vi "DI sensor handling full_ext.vi"(0 "DI":bool, 1 "SOURCE":u32=1 max=2 step=1, 2 "SOURCE_ALLOW":bool, 3 "DI2":bool, 4 "control":cluster{"invert":dbl, "time_const":dbl}={"invert"=1.0, "time_const"=100.0} {"time_const" min=1.0 max=100000.0 step=1.0}, 6 "initialise":bool, 7 "DI sensor handling full reg old":T2 {"RS32 Q" format="%x"}, 8 "connect":bool) -> (13 "DI sensor handling full reg":T1 {"RS32 Q" format="%x"}, 14 "DIOUT":bool caption="PVOUT", 15 "SOURCEOUT":u32=1 max=2 step=1, 16 "STATE":T3, 17 "block":u32 format="%09b", 19 "ALRSTATE":errorcluster)   [LabVIEW 2019, in "Inputs.lvlib"]
uses:
  Inputs.lvlib
  Ctl/Parameter State.ctl
  Ctl/Sensor alarm.ctl
  Ctl/Sensor state.ctl
  Trigers/RS_ext.vi
  Logik/Logik.lvlib
  Trigers/Triggers.lvlib
  Timer Delay/Timers.lvlib
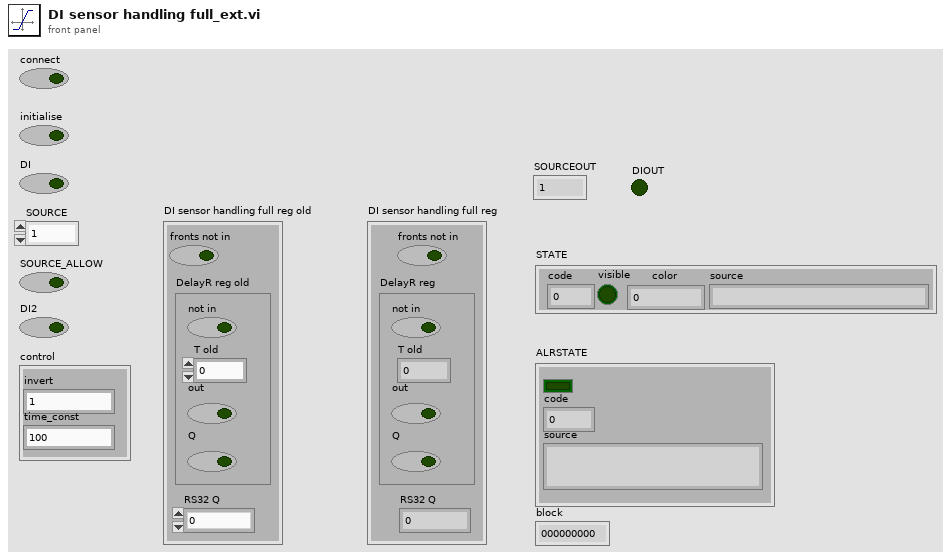
[diagram p1: front panel]
types:
  T1 = cluster{"fronts not in":bool, "DelayR reg":cluster{"not in":bool, "T old":u32, "out":bool, "Q":bool}, "RS32 Q":u32}
  T2 = cluster{"fronts not in":bool, "DelayR reg old":cluster{"not in":bool, "T old":u32, "out":bool, "Q":bool}, "RS32 Q":u32}
  T3 = typedef "Inputs.lvlib/Parameter State.ctl" = cluster{"code":i32, "visible":bool, "color":u32, "source":string}
  T4 = typedef "Inputs.lvlib/Sensor alarm.ctl" = cluster{"source":string, "color":u32, "visible":bool}[]
  T5 = typedef "Inputs.lvlib/Sensor state.ctl" = cluster{"source":string, "color":u32, "visible":bool}[]
  T6 = cluster{"not in":bool, "T old":u32, "out":bool, "Q":bool}
  T7 = cluster{"source":string, "color":u32, "visible":bool}
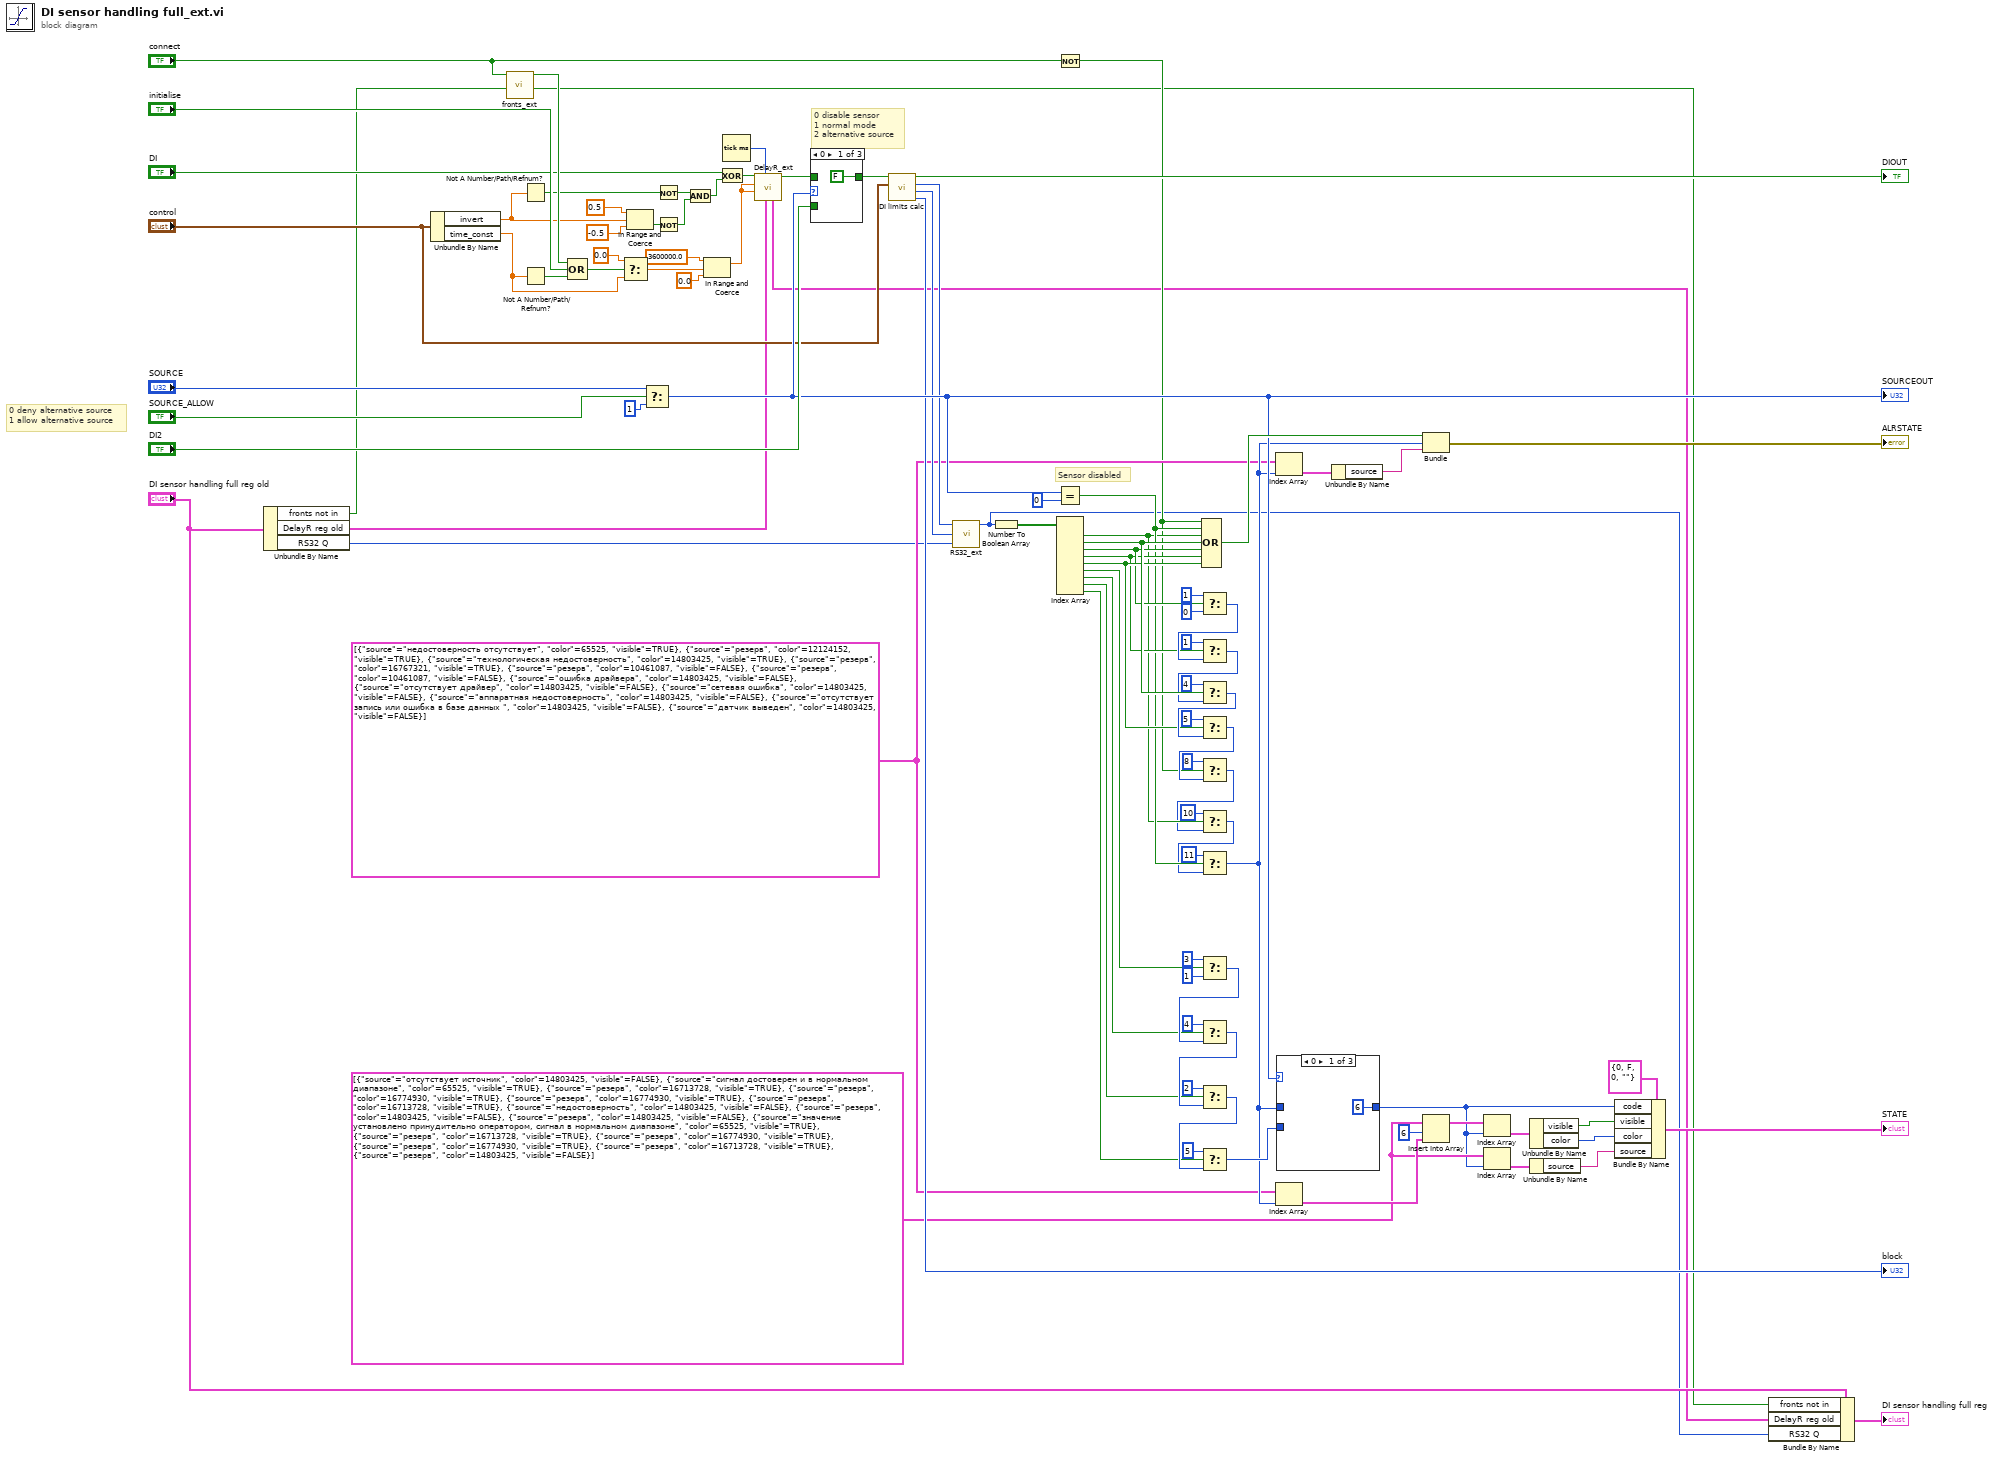
[diagram p0: block diagram]
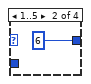
[diagram p5: hidden frame]
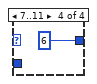
[diagram p7: hidden frame]
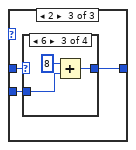
[diagram p8: hidden frame]
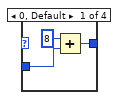
[diagram p9: hidden frame]
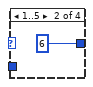
[diagram p10: hidden frame]
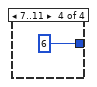
[diagram p11: hidden frame]
diagram:
  w39 = T4 [{"source"="недостоверность отсутствует", "color"=65525, "visible"=TRUE}, {"source"="резерв", "color"=12124152, "visible"=TRUE}, {"source"="технологическая недостоверность", "color"=14803425, "visible"=TRUE}, {"source"="резерв", "color"=16767321, "visible"=TRUE}, {"source"="резерв", "color"=10461087, "visible"=FALSE}, {"source"="резерв", "color"=10461087, "visible"=FALSE}, {"source"="ошибка драйвера", "color"=14803425, "visible"=FALSE}, {"source"="отсутствует драйвер", "color"=14803425, "visible"=FALSE}, {"source"="сетевая ошибка", "color"=14803425, "visible"=FALSE}, {"source"="аппаратная недостоверность", "color"=14803425, "visible"=FALSE}, {"source"="отсутствует запись или ошибка в базе данных ", "color"=14803425, "visible"=FALSE}, {"source"="датчик выведен", "color"=14803425, "visible"=FALSE}]
  w47 = T5 [{"source"="отсутствует источник", "color"=14803425, "visible"=FALSE}, {"source"="сигнал достоверен и в нормальном диапазоне", "color"=65525, "visible"=TRUE}, {"source"="резерв", "color"=16713728, "visible"=TRUE}, {"source"="резерв", "color"=16774930, "visible"=TRUE}, {"source"="резерв", "color"=16774930, "visible"=TRUE}, {"source"="резерв", "color"=16713728, "visible"=TRUE}, {"source"="недостоверность", "color"=14803425, "visible"=FALSE}, {"source"="резерв", "color"=14803425, "visible"=FALSE}, {"source"="резерв", "color"=14803425, "visible"=FALSE}, {"source"="значение установлено принудительно оператором, сигнал в нормальном диапазоне", "color"=65525, "visible"=TRUE}, {"source"="резерв", "color"=16713728, "visible"=TRUE}, {"source"="резерв", "color"=16774930, "visible"=TRUE}, {"source"="резерв", "color"=16774930, "visible"=TRUE}, {"source"="резерв", "color"=16713728, "visible"=TRUE}, {"source"="резерв", "color"=14803425, "visible"=FALSE}]
  # "Sensor disabled"
  # "0 disable sensor\n1 normal mode\n2 alternative source"
  # "0 deny alternative source\n1 allow alternative source"
  n1 = Unbundle By Name("DI sensor handling full reg old") -> ("fronts not in"=w11:bool, "DelayR reg old"=w9:T6, "RS32 Q"=w8:u32)
  n2 = Unbundle By Name("control") -> ("invert"=w18:dbl, "time_const"=w29:dbl)
  n3 = call "fronts_ext.vi"("not in old"=w11, "in"="connect") -> ("not in"=w12:bool, "raise"=w36:bool)  [unwired: 3 in, 1 out]
  n4 = Not A Number/Path/Refnum?(number/path/refnum=w18) -> (NaN/Path/Refnum?=w17:bool)
  n5 = Not A Number/Path/Refnum?(number/path/refnum=w29) -> (NaN/Path/Refnum?=w20:bool)
  n6 = Compound Arithmetic op=OR(w36, "initialise", w20) -> (w19:bool)
  n7 = Select(t=0.0, s=w19, f=w29) -> (s? t:f=w25:dbl)
  n8 = In Range and Coerce(upper limit=0.5, x=w18, lower limit=-0.5 ("upper limit")) -> (In Range?=w23:bool)  [unwired: 1 out]
  n9 = Select(t="SOURCE", s="SOURCE_ALLOW", f=u32 1) -> (s? t:f=w72:u32)
  "SOURCEOUT" <- w72
  n10 = Not(x=w17) -> (.not. x?=w16:bool)
  n11 = Not(x=w23) -> (.not. x?=w15:bool)
  n12 = And(x=w16, y=w15) -> (x .and. y?=w14:bool)
  n13 = In Range and Coerce(upper limit=3600000.0, x=w25, lower limit=0.0 ("upper limit")) -> (coerced(x)=w24:dbl)  [unwired: 1 out]
  n14 = Exclusive Or(1:w14, 2:"DI") -> (0:w21:bool)
  n15 = Tick Count (ms)() -> (millisecond timer value=w1:u32)
  n16 = call "DelayR_ext.vi"("DelayR reg old"=w9, "T  ms (0 curr)"=w1, "DelayOff (0)"=w24, "DelayOn (0)"=w24, "In"=w21) -> ("Out"=w34:bool, "DelayR reg"=w6:T6)  [unwired: 4 in, 1 out]
  n17 = case shown="0" w72 {
    tunnel: w34 -> [_ w98 _]
    tunnel: [FALSE w98 w99] -> w31
    tunnel: "DI2" -> [_ _ w99]
    frame 0 {
    }
    frame 1, Default {
    }
    frame 2 {
    }
  }
  n18 = call "DI limits calc.vi"("control"="control", "DI"=w31) -> ("block"=→"block":u32, "Off"=w57:u32, "On"=w58:u32, "DIOUT"=→"DIOUT":bool)  [unwired: 2 in]
  n19 = call "RS32_ext.vi"("Q old"=w8, "R"=w57, "S"=w58) -> ("Q"=w7:u32)  [unwired: 1 in, 1 out]
  n20 = Number To Boolean Array(number=w7) -> (Boolean array=w77:bool[])
  n21 = Not(x="connect") -> (.not. x?=w37:bool)
  n22 = Equal?(x=w72, y=u32 0) -> (x = y?=w61:bool)
  n23 = Index Array(array=w77) -> (element #1=w59:bool, element #2=w76:bool, element #3=w63:bool, element #4=w62:bool, element #5=w67:bool, element #6=w68:bool, element #7=w69:bool, element #8=w70:bool, element #9=w71:bool)  [unwired: 9 in]
  n24 = Compound Arithmetic op=OR ("status")(w37, w61, w59, w76, w63, w62, w67) -> (w82:bool)
  n25 = Select ("code")(t=1, s=w63, f=0) -> (s? t:f=w65:i32)
  n26 = Select ("code")(t=1, s=w62, f=w65) -> (s? t:f=w64:i32)
  n27 = Select ("code")(t=4, s=w76, f=w64) -> (s? t:f=w91:i32)
  n28 = Select ("code")(t=5, s=w67, f=w91) -> (s? t:f=w42:i32)
  n29 = Select ("code")(t=8, s=w37, f=w42) -> (s? t:f=w41:i32)
  n30 = Select ("code")(t=10, s=w59, f=w41) -> (s? t:f=w48:i32)
  n31 = Select ("code")(t=11, s=w61, f=w48) -> (s? t:f=w53:i32)
  n32 = Select ("code")(t=3 ("code"), s=w68, f=1 ("code")) -> (s? t:f=w86:i32)
  n33 = Select ("code")(t=4 ("code"), s=w69, f=w86) -> (s? t:f=w85:i32)
  n34 = Select ("code")(t=2 ("code"), s=w70, f=w85) -> (s? t:f=w83:i32)
  n35 = Select ("code")(t=5 ("code"), s=w71, f=w83) -> (s? t:f=w78:i32)
  n36 = Index Array(array=w39, index=w53) -> (element=w51:T7)
  n37 = Index Array(array=w39, index=w53) -> (element=w50:T7)
  n38 = case "code" shown="0" w72 {
    tunnel: w53 -> [_ w103 w110]
    tunnel: w78 -> [_ w102 w109]
    tunnel: [6 ("code") w101 w108] -> w45
    frame 0 {
    }
    frame 1, Default {
      n39 = case "code" shown="0, Default" w103 {
        tunnel: [w104 6 ("code") w106 6 ("code")] -> w101
        tunnel: w102 -> [w104 _ w106 _]
        frame 0, Default {
        }
        frame 1..5 {
        }
        frame 6 {
        }
        frame 7..11 {
        }
      }
    }
    frame 2 {
      n40 = case "code" shown="6" w110 {
        tunnel: [w112 6 ("code") w116 6 ("code")] -> w108
        tunnel: w109 -> [w113 _ w115 _]
        frame 0, Default {
          n41 = Add ("code")(x=8 ("code"), y=w113) -> (x+y=w112:i32)
        }
        frame 1..5 {
        }
        frame 6 {
          n42 = Add ("code")(x=8 ("code"), y=w115) -> (x+y=w116:i32)
        }
        frame 7..11 {
        }
      }
    }
  }
  n43 = Unbundle By Name(w51) -> ("source"=w52:string)
  n44 = Bundle(w82, w53, "source"=w52) -> (→"ALRSTATE":cluster{bool, i32, "source":string})  [unwired: 1 in]
  n45 = Insert Into Array(array=w47, index=6, new element=w50) -> (w54:T5)
  n46 = Index Array(array=w54, index=w45) -> (element=w49:T7)
  n47 = Index Array(array=w47, index=w45) -> (element=w46:T7)
  n48 = Unbundle By Name(w49) -> ("visible"=w4:bool, "color"=w3:u32)
  n49 = Unbundle By Name(w46) -> ("source"=w2:string)
  n50 = Bundle By Name(cluster=T3 {"code"=0, "visible"=FALSE, "color"=0, "source"=""} ("STATE"), "code"=w45, "visible"=w4, "color"=w3, "source"=w2) -> (→"STATE":T3)
  n51 = Bundle By Name(cluster="DI sensor handling full reg old", "fronts not in"=w12, "DelayR reg old"=w6, "RS32 Q"=w7) -> (→"DI sensor handling full reg":T2)
